vi "LoadINIFile.vi"(8 "error in":errorcluster, 11 "Sequence Context In":refnum<k7>) -> (0 "error out":errorcluster)   [LabVIEW 2021]
uses:
  <vilib>/Utility/config.llb/Read Key (String).vi
  <vilib>/addons/TestStand/_TSUtility.llb/TestStand - Set Property Value (String).vi
  <vilib>/addons/TestStand/_TSUtility.llb/TestStand - Set Property Value (Number).vi
  <vilib>/Utility/config.llb/NI_LVConfig.lvlib
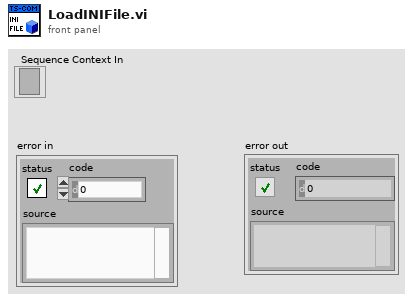
[diagram p1: front panel]
types:
  T1 = typedef "NI_LVConfig.lvlib/Config Data RefNum.ctl" = refnum<k1>
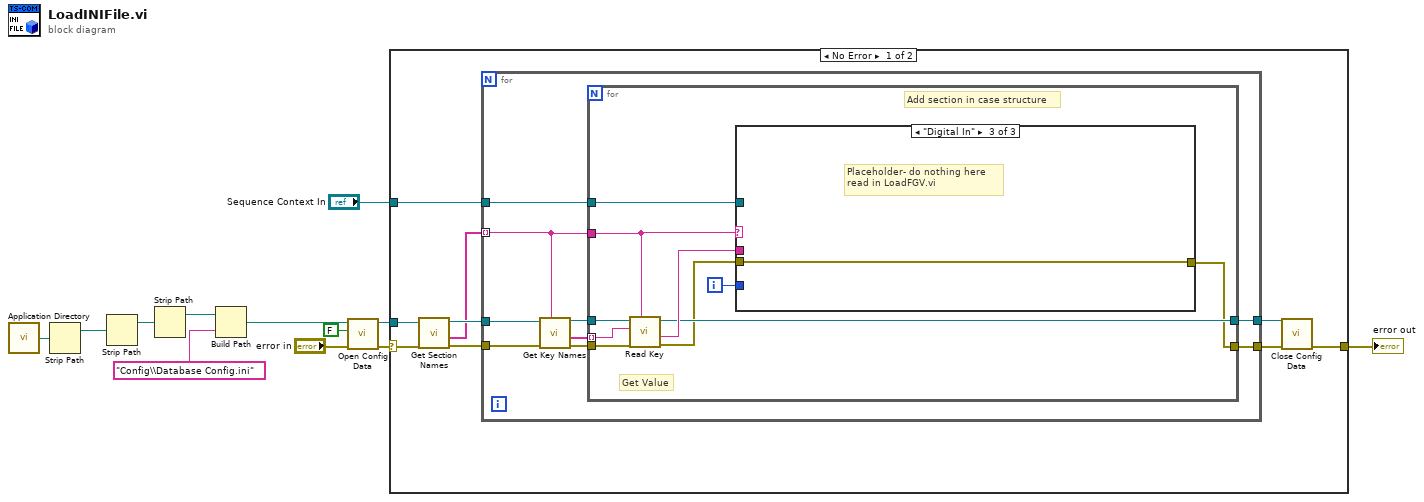
[diagram p0: block diagram]
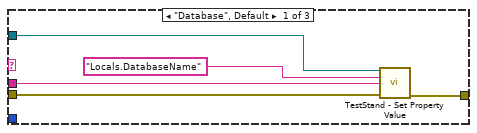
[diagram p2: hidden frame]
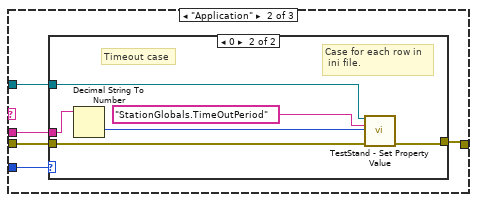
[diagram p3: hidden frame]
diagram:
  n1 = call <vilib>:"Application Directory.vi"() -> ("Application Directory"=w12:path)
  n2 = Strip Path(path=w12) -> (stripped path=w11:path)  [unwired: 1 out]
  n3 = Strip Path(path=w11) -> (stripped path=w2:path)  [unwired: 1 out]
  n4 = Strip Path(path=w2) -> (stripped path=w1:path)  [unwired: 1 out]
  n5 = Build Path(base path=w1, name or relative path="Config\\Database Config.ini") -> (appended path=w8:path)
  n6 = call <vilib>:"Open Config Data.vi"("error in (no error)"="error in", "create file if necessary (T)"=FALSE, "configuration file path"=w8) -> ("error out"=w5:errorcluster, "refnum"=w6:T1)  [unwired: 6 in, 1 out]
  n7 = case shown="No Error" w5 {
    selector: w5 -> [w18 w59]
    tunnel: w6 -> [w21 _]
    tunnel: "Sequence Context In" -> [w14 _]
    tunnel: [w13 w59] -> w3
    frame No Error {
      n8 = call <vilib>:"Get Section Names.vi"("error in (no error)"=w18, "refnum"=w21) -> ("error out"=w20:errorcluster, "section names"=w17:string[], "refnum out"=w19:T1)  [unwired: 7 in]
      n9 = for {
        tunnel: w20 -> [w30]
        tunnel: w19 -> [w29]
        tunnel: w17 -> [w25] mode=indexing
        tunnel: [w24] -> w16
        tunnel: [w23] -> w15
        tunnel: w14 -> [w22]
        n10 = call <vilib>:"Get Key Names.vi"("section"=w25, "error in (no error)"=w30, "refnum"=w29) -> ("error out"=w27:errorcluster, "key names"=w28:string[], "refnum out"=w26:T1)  [unwired: 5 in, 1 out]
        n11 = for {
          tunnel: w28 -> [w39] mode=indexing
          tunnel: w27 -> [w40]
          tunnel: w26 -> [w38]
          tunnel: w25 -> [w37]
          tunnel: [w32] -> w24
          tunnel: [w35] -> w23
          tunnel: w22 -> [w34]
          i -> [w31]
          # "Add section in case structure"
          # "Get Value"
          n12 = call-poly <vilib>:"Read Key.vi"("section"=w37, "error in (no error)"=w40, "key"=w39, "refnum"=w38) -> ("error out"=w33:errorcluster, "value"=w36:string, "refnum out"=w35:T1)  [unwired: 4 in, 1 out]
          n13 = case shown="\"Digital In\"" w37 {
            tunnel: w36 -> [w45 w48 _]
            tunnel: w34 -> [w41 w49 _]
            tunnel: w33 -> [w44 w50 w58]
            tunnel: [w42 w46 w58] -> w32
            tunnel: w31 -> [_ w47 _]
            frame "Database", Default {
              n14 = call-poly <vilib>:"TestStand - Set Property Value.vi"("Sequence Context In"=w41, "Lookup String"="Locals.DatabaseName", "New Value"=w45, "error in (no error)"=w44) -> ("error out"=w42:errorcluster)  [unwired: 10 in, 1 out]
            }
            frame "Application" {
              n15 = case shown="0" w47 {
                tunnel: w50 -> [w51 w57]
                tunnel: w49 -> [_ w55]
                tunnel: w48 -> [_ w54]
                tunnel: [w51 w52] -> w46
                frame -1, Default {
                }
                frame 0 {
                  # "Timeout case"
                  # "Case for each row in\n ini file."
                  n16 = Decimal String To Number(string=w54) -> (number=w53:i32)  [unwired: 2 in, 1 out]
                  n17 = call-poly <vilib>:"TestStand - Set Property Value.vi"("Sequence Context In"=w55, "Lookup String"="StationGlobals.TimeOutPeriod", "New Value"=w53, "error in (no error)"=w57) -> ("error out"=w52:errorcluster)  [unwired: 10 in, 1 out]
                }
              }
            }
            frame "Digital In" {
              # "Placeholder- do nothing here\nread in LoadFGV.vi"
            }
          }
        }
      }
      n18 = call <vilib>:"Close Config Data.vi"("error in (no error)"=w16, "refnum"=w15) -> ("error out"=w13:errorcluster)  [unwired: 8 in, 1 out]
    }
    frame Error {
    }
  }
  "error out" <- w3
